vi "lorentzian transformations--test.vi"() -> ()   [LabVIEW 2020]
uses:
  lorentzian.ctl
  circle corners.ctl
  cursor action.ctl
  four-corner circle transformation.ctl
  draw a circle.vi
  draw a complex arrow.vi
  Q -- check range -- i -- real.vi
  generate linear region.vi
  draw a complex line.vi
  Q - not nan -- real.vi
panel:
  in  "Tab Control":enum32{"Page 1", "Page 2"}(tab)
  in  "phase0":dbl(slide)=-0.3274811506911865 scale=-1.57..1.57
  in  "factor":dbl(slide)=0.3 scale=-3.0..3.0
  in  "phase":dbl(slide)=-0.2854545454545454 scale=-1.57..1.57
  out "Plot: complex plane":cluster{dbl[], dbl[]}[](graph)=[{[1.005, 1.0049956141504943, 1.0049824642962475, 1.0049605735065723, 1.0049299801853526, 1.0048907380036691, 1.004842915805643, 1.0047865974876604, 1.0047218818511874, 1.0046488824294413, 1.004567727288213, 1.004478558801197, 1.0043815334002193, 1.0042768213008024, 1.0041646062035505, 1.0040450849718747, 1.0039184672866293, 1.0037849752782588, 1.003644843137107, 1.0034983167025668, 1.0033456530317943, 1.0031871199487434, 1.003022995574312, 1.002853567838422, 1.002679133974895, 1.0025, 1.0023164801755993, 1.0021288964578254, 1.0019375779322606, 1.001742860236609, 1.0015450849718748, 1.0013445991030763, 1.0011417543505532, 1.0009369065729286, 1.000730415142812, 1.0005226423163383, 1.0003139525976465, 1.0001047120994169, 0.9998952879005832, 0.9996860474023535, 0.9994773576836617, 0.999269584857188, 0.9990630934270713, 0.9988582456494467, 0.9986554008969236, 0.9984549150281252, 0.9982571397633909, 0.9980624220677395, 0.9978711035421747, 0.9976835198244007, 0.9975, 0.9973208660251051, 0.9971464321615778, 0.9969770044256882, 0.9968128800512566, 0.9966543469682058, 0.9965016832974332, 0.996355156862893, 0.9962150247217412, 0.9960815327133709, 0.9959549150281253, 0.9958353937964495, 0.9957231786991975, 0.9956184665997807, 0.9955214411988029, 0.995432272711787, 0.9953511175705587, 0.9952781181488126, 0.9952134025123397, 0.9951570841943569, 0.995109261996331, 0.9950700198146475, 0.9950394264934276, 0.9950175357037525, 0.9950043858495057, 0.995, 0.9950043858495057, 0.9950175357037525, 0.9950394264934276, 0.9950700198146475, 0.995109261996331, 0.9951570841943569, 0.9952134025123397, 0.9952781181488126, 0.9953511175705587, 0.995432272711787, 0.9955214411988029, 0.9956184665997807, 0.9957231786991975, 0.9958353937964495, 0.9959549150281253, 0.9960815327133709, 0.9962150247217412, 0.9963551568628929, 0.9965016832974332, 0.9966543469682058, 0.9968128800512566, 0.9969770044256882, 0.9971464321615778, 0.9973208660251051, 0.9975, 0.9976835198244007, 0.9978711035421747, 0.9980624220677394, 0.9982571397633909, 0.9984549150281252, 0.9986554008969236, 0.9988582456494467, 0.9990630934270713, 0.999269584857188, 0.9994773576836617, 0.9996860474023535, 0.9998952879005832, 1.0001047120994169, 1.0003139525976465, 1.0005226423163383, 1.000730415142812, 1.0009369065729286, 1.0011417543505532, 1.0013445991030763, 1.0015450849718748, 1.001742860236609, 1.0019375779322606, 1.0021288964578254, 1.0023164801755993, 1.0025, 1.002679133974895, 1.002853567838422, 1.003022995574312, 1.0031871199487434, 1.0033456530317943, 1.0034983167025668, 1.003644843137107, 1.0037849752782588, 1.0039184672866293, 1.0040450849718747, 1.0041646062035505, 1.0042768213008024, 1.0043815334002193, 1.004478558801197, 1.004567727288213, 1.0046488824294413, 1.0047218818511874, 1.0047865974876604, 1.004842915805643, 1.0048907380036691, 1.0049299801853526, 1.0049605735065723, 1.0049824642962475, 1.0049956141504943], [0.995, 0.995209378268646, 0.9954183892166616, 0.9956266661678215, 0.9958338437335805, 0.9960395584540888, 0.9962434494358243, 0.9964451589847223, 0.996644333233693, 0.9968406227634233, 0.997033683215379, 0.9972231758959247, 0.9974087683705086, 0.9975901350468657, 0.9977669577462167, 0.9979389262614624, 0.9981057389013915, 0.9982671030199505, 0.9984227355296434, 0.998572363398164, 0.998715724127387, 0.998852566213879, 0.998982649590121, 0.9991057460456685, 0.9992216396275101, 0.9993301270189222, 0.9994310178961561, 0.9995241352623301, 0.9996093157579425, 0.9996864099474595, 0.9997552825814757, 0.9998158128339882, 0.9998678945143658, 0.9999114362536434, 0.999946361664815, 0.9999726094768414, 0.9999901336421414, 0.9999989034173742, 0.9999989034173742, 0.9999901336421414, 0.9999726094768414, 0.999946361664815, 0.9999114362536434, 0.9998678945143658, 0.9998158128339882, 0.9997552825814757, 0.9996864099474595, 0.9996093157579425, 0.9995241352623301, 0.9994310178961561, 0.9993301270189222, 0.9992216396275101, 0.9991057460456685, 0.998982649590121, 0.998852566213879, 0.998715724127387, 0.998572363398164, 0.9984227355296434, 0.9982671030199505, 0.9981057389013915, 0.9979389262614624, 0.9977669577462167, 0.9975901350468657, 0.9974087683705086, 0.9972231758959247, 0.997033683215379, 0.9968406227634233, 0.996644333233693, 0.9964451589847223, 0.9962434494358243, 0.9960395584540888, 0.9958338437335805, 0.9956266661678215, 0.9954183892166616, 0.995209378268646, 0.995, 0.994790621731354, 0.9945816107833384, 0.9943733338321785, 0.9941661562664195, 0.9939604415459112, 0.9937565505641758, 0.9935548410152777, 0.993355666766307, 0.9931593772365767, 0.992966316784621, 0.9927768241040753, 0.9925912316294914, 0.9924098649531343, 0.9922330422537833, 0.9920610737385376, 0.9918942610986085, 0.9917328969800495, 0.9915772644703565, 0.991427636601836, 0.991284275872613, 0.991147433786121, 0.991017350409879, 0.9908942539543315, 0.9907783603724899, 0.9906698729810778, 0.9905689821038439, 0.9904758647376699, 0.9903906842420575, 0.9903135900525405, 0.9902447174185243, 0.9901841871660118, 0.9901321054856342, 0.9900885637463566, 0.990053638335185, 0.9900273905231586, 0.9900098663578586, 0.9900010965826258, 0.9900010965826258, 0.9900098663578586, 0.9900273905231586, 0.990053638335185, 0.9900885637463566, 0.9901321054856342, 0.9901841871660118, 0.9902447174185243, 0.9903135900525405, 0.9903906842420575, 0.9904758647376699, 0.9905689821038439, 0.9906698729810778, 0.9907783603724899, 0.9908942539543315, 0.991017350409879, 0.991147433786121, 0.991284275872613, 0.991427636601836, 0.9915772644703565, 0.9917328969800495, 0.9918942610986085, 0.9920610737385376, 0.9922330422537833, 0.9924098649531343, 0.9925912316294914, 0.9927768241040753, 0.992966316784621, 0.9931593772365767, 0.993355666766307, 0.9935548410152777, 0.9937565505641757, 0.9939604415459112, 0.9941661562664195, 0.9943733338321785, 0.9945816107833384, 0.994790621731354]}, {[1.0, 1.0, 1.0, 1.0, 1.0, 1.0, 1.0, 1.0, 1.0, 1.0, 1.0, 1.0, 1.0, 1.0, 1.0, 1.0, 1.0, 1.0, 1.0, 1.0], [1.0, 0.9995, 0.999, 0.9984999999999999, 0.998, 0.9975, 0.997, 0.9964999999999999, 0.996, 0.9955, 0.995, 0.9944999999999999, 0.994, 0.9935, 0.993, 0.9924999999999999, 0.992, 0.9915, 0.991, 0.9904999999999999]}, {[1.005, 1.0045, 1.004, 1.0034999999999998, 1.003, 1.0025, 1.002, 1.0014999999999998, 1.001, 1.0005, 1.0, 0.9994999999999999, 0.999, 0.9984999999999999, 0.998, 0.9974999999999999, 0.997, 0.9964999999999999, 0.996, 0.9954999999999999], [0.995, 0.995, 0.995, 0.995, 0.995, 0.995, 0.995, 0.995, 0.995, 0.995, 0.995, 0.995, 0.995, 0.995, 0.995, 0.995, 0.995, 0.995, 0.995, 0.995]}, {[1.01, 1.009, 1.008, 1.0070000000000001, 1.006, 1.005, 1.004, 1.0030000000000001, 1.002, 1.001, 1.0, 0.999, 0.998, 0.997, 0.996, 0.995, 0.994, 0.993, 0.992, 0.991], [1.0, 1.0, 1.0, 1.0, 1.0, 1.0, 1.0, 1.0, 1.0, 1.0, 1.0, 1.0, 1.0, 1.0, 1.0, 1.0, 1.0, 1.0, 1.0, 1.0]}, {[1.0059232929877608, 1.0059187898532358, 1.0059052883496888, 1.005882812163345, 1.0058514007250723, 1.0058111091412076, 1.0057620080968799, 1.0057041837320058, 1.00563773749017, 1.005562785940659, 1.0054794605739599, 1.0053879075710797, 1.0052882875470954, 1.0051807752693802, 1.0050655593510023, 1.0049428419198327, 1.0048128382639459, 1.0046757764539296, 1.0045318969427723, 1.0043814521440277, 1.0042247059889937, 1.0040619334636893, 1.003893420126434, 1.003719461606883, 1.003540363087391, 1.0033564387676188, 1.003168011313322, 1.0029754112902827, 1.0027789765843875, 1.00257905180886, 1.0023759876996907, 1.0021701405003292, 1.00196187133671, 1.0017515455837172, 1.00153953222419, 1.001326203201604, 1.0011119327675542, 1.000897096825192, 1.0006820722697616, 1.0004672363273994, 1.0002529658933497, 1.0000396368707636, 0.9998276235112366, 0.9996172977582435, 0.9994090285946245, 0.9992031813952629, 0.9990001172860937, 0.998800192510566, 0.998603757804671, 0.9984111577816318, 0.9982227303273348, 0.9980388060075627, 0.9978597074880705, 0.9976857489685195, 0.9975172356312644, 0.9973544631059599, 0.997197716950926, 0.9970472721521811, 0.996903392641024, 0.9967663308310076, 0.9966363271751209, 0.9965136097439514, 0.9963983938255734, 0.9962908815478583, 0.9961912615238739, 0.9960997085209937, 0.9960163831542945, 0.9959414316047838, 0.9958749853629478, 0.9958171609980736, 0.995768059953746, 0.9957277683698812, 0.9956963569316087, 0.9956738807452647, 0.9956603792417177, 0.9956558761071926, 0.9956603792417177, 0.9956738807452647, 0.9956963569316087, 0.9957277683698812, 0.995768059953746, 0.9958171609980736, 0.9958749853629478, 0.9959414316047838, 0.9960163831542945, 0.9960997085209937, 0.9961912615238739, 0.9962908815478583, 0.9963983938255734, 0.9965136097439514, 0.9966363271751209, 0.9967663308310076, 0.996903392641024, 0.9970472721521811, 0.997197716950926, 0.9973544631059599, 0.9975172356312644, 0.9976857489685195, 0.9978597074880705, 0.9980388060075627, 0.9982227303273348, 0.9984111577816318, 0.998603757804671, 0.998800192510566, 0.9990001172860937, 0.9992031813952629, 0.9994090285946245, 0.9996172977582435, 0.9998276235112366, 1.0000396368707636, 1.0002529658933497, 1.0004672363273994, 1.0006820722697616, 1.000897096825192, 1.0011119327675542, 1.001326203201604, 1.00153953222419, 1.0017515455837172, 1.00196187133671, 1.0021701405003292, 1.0023759876996907, 1.00257905180886, 1.0027789765843875, 1.0029754112902827, 1.003168011313322, 1.0033564387676188, 1.003540363087391, 1.003719461606883, 1.003893420126434, 1.0040619334636893, 1.0042247059889937, 1.0043814521440277, 1.0045318969427723, 1.0046757764539296, 1.0048128382639459, 1.0049428419198327, 1.005065559351002, 1.0051807752693802, 1.0052882875470954, 1.0053879075710797, 1.0054794605739599, 1.005562785940659, 1.00563773749017, 1.0057041837320058, 1.0057620080968799, 1.0058111091412076, 1.0058514007250723, 1.005882812163345, 1.0059052883496888, 1.0059187898532358], [0.994938915988178, 0.99515389338517, 0.9953684936387578, 0.9955823402671752, 0.9957950581107701, 0.9960062739901628, 0.9962156173609295, 0.9964227209636622, 0.9966272214682678, 0.9968287601113711, 0.997026983325709, 0.9972215433604069, 0.9974120988910519, 0.997598315618492, 0.9977798668553104, 0.9979564340989464, 0.9981277075904564, 0.9982933868579376, 0.9984531812436561, 0.9986068104139613, 0.9987540048510848, 0.9988945063259668, 0.9990280683512777, 0.9991544566138403, 0.9992734493856953, 0.9993848379130866, 0.9994884267826872, 0.9995840342644202, 0.9996714926302748, 0.9997506484485588, 0.9998213628530697, 0.9998835117867129, 0.9999369862191405, 0.9999816923380274, 1.0000175517136496, 1.0000445014364774, 1.0000624942275393, 1.000071498521366, 1.000071498521366, 1.0000624942275393, 1.0000445014364774, 1.0000175517136496, 0.9999816923380274, 0.9999369862191405, 0.9998835117867129, 0.9998213628530697, 0.9997506484485588, 0.9996714926302748, 0.9995840342644202, 0.9994884267826872, 0.9993848379130866, 0.9992734493856953, 0.9991544566138403, 0.9990280683512777, 0.9988945063259668, 0.9987540048510848, 0.9986068104139613, 0.9984531812436561, 0.9982933868579376, 0.9981277075904564, 0.9979564340989464, 0.9977798668553104, 0.997598315618492, 0.9974120988910519, 0.9972215433604069, 0.997026983325709, 0.9968287601113711, 0.9966272214682678, 0.9964227209636622, 0.9962156173609295, 0.9960062739901628, 0.9957950581107701, 0.9955823402671752, 0.9953684936387579, 0.99515389338517, 0.994938915988178, 0.9947239385911859, 0.9945093383375981, 0.9942954917091807, 0.9940827738655859, 0.9938715579861931, 0.9936622146154265, 0.9934551110126937, 0.9932506105080882, 0.9930490718649848, 0.9928508486506469, 0.992656288615949, 0.9924657330853041, 0.9922795163578639, 0.9920979651210455, 0.9919213978774095, 0.9917501243858995, 0.9915844451184184, 0.9914246507326998, 0.9912710215623947, 0.9911238271252711, 0.9909833256503892, 0.9908497636250783, 0.9907233753625156, 0.9906043825906606, 0.9904929940632693, 0.9903894051936687, 0.9902937977119357, 0.9902063393460812, 0.9901271835277972, 0.9900564691232863, 0.9899943201896431, 0.9899408457572154, 0.9898961396383286, 0.9898602802627063, 0.9898333305398784, 0.9898153377488166, 0.9898063334549901, 0.9898063334549901, 0.9898153377488166, 0.9898333305398784, 0.9898602802627063, 0.9898961396383286, 0.9899408457572154, 0.9899943201896431, 0.9900564691232863, 0.9901271835277972, 0.9902063393460812, 0.9902937977119357, 0.9903894051936687, 0.9904929940632693, 0.9906043825906606, 0.9907233753625156, 0.9908497636250783, 0.9909833256503892, 0.9911238271252711, 0.9912710215623947, 0.9914246507326998, 0.9915844451184184, 0.9917501243858995, 0.9919213978774095, 0.9920979651210455, 0.9922795163578639, 0.9924657330853041, 0.992656288615949, 0.9928508486506469, 0.9930490718649848, 0.9932506105080882, 0.9934551110126937, 0.9936622146154265, 0.9938715579861931, 0.9940827738655859, 0.9942954917091807, 0.994509338337598, 0.9947239385911859]}, {[1.0007895845474768, 1.0007895845474768, 1.0007895845474768, 1.0007895845474768, 1.0007895845474768, 1.0007895845474768, 1.0007895845474768, 1.0007895845474768, 1.0007895845474768, 1.0007895845474768, 1.0007895845474768, 1.0007895845474768, 1.0007895845474768, 1.0007895845474768, 1.0007895845474768, 1.0007895845474768, 1.0007895845474768, 1.0007895845474768, 1.0007895845474768, 1.0007895845474768], [1.0000726244284621, 0.9995592535844338, 0.9990458827404053, 0.9985325118963768, 0.9980191410523485, 0.9975057702083201, 0.9969923993642916, 0.9964790285202632, 0.9959656576762348, 0.9954522868322064, 0.994938915988178, 0.9944255451441495, 0.9939121743001211, 0.9933988034560928, 0.9928854326120643, 0.9923720617680358, 0.9918586909240075, 0.9913453200799791, 0.9908319492359506, 0.9903185783919222]}, {[1.0059232929877608, 1.0054099221437325, 1.0048965512997041, 1.0043831804556755, 1.0038698096116472, 1.0033564387676188, 1.0028430679235905, 1.0023296970795619, 1.0018163262355335, 1.0013029553915052, 1.0007895845474768, 1.0002762137034484, 0.99976284285942, 0.9992494720153915, 0.9987361011713631, 0.9982227303273347, 0.9977093594833063, 0.9971959886392778, 0.9966826177952495, 0.996169246951221], [0.994938915988178, 0.994938915988178, 0.994938915988178, 0.994938915988178, 0.994938915988178, 0.994938915988178, 0.994938915988178, 0.994938915988178, 0.994938915988178, 0.994938915988178, 0.994938915988178, 0.994938915988178, 0.994938915988178, 0.994938915988178, 0.994938915988178, 0.994938915988178, 0.994938915988178, 0.994938915988178, 0.994938915988178, 0.994938915988178]}, {[1.011057001428045, 1.0100302597399882, 1.0090035180519314, 1.0079767763638747, 1.0069500346758178, 1.0059232929877608, 1.0048965512997041, 1.0038698096116474, 1.0028430679235905, 1.0018163262355335, 1.0007895845474768, 0.99976284285942, 0.9987361011713631, 0.9977093594833063, 0.9966826177952495, 0.9956558761071926, 0.9946291344191358, 0.993602392731079, 0.9925756510430221, 0.9915489093549653], [1.0000726244284621, 1.0000726244284621, 1.0000726244284621, 1.0000726244284621, 1.0000726244284621, 1.0000726244284621, 1.0000726244284621, 1.0000726244284621, 1.0000726244284621, 1.0000726244284621, 1.0000726244284621, 1.0000726244284621, 1.0000726244284621, 1.0000726244284621, 1.0000726244284621, 1.0000726244284621, 1.0000726244284621, 1.0000726244284621, 1.0000726244284621, 1.0000726244284621]}]
  in  "lorentzian":T1={"A (VHz)"=1.0, "f (Hz)"=900.0, "G (Hz)"=200.0, "phi(rad)"=0.0, "Q"=0.006429595340103388, "Norm  Ampl"=nan, "bg (V)"=1.0+1.0i, "4corners"={"z (-pi/2)"=1.005+0.995i, "z(inf)"=1.0+1.0i, "z (pi/2)"=0.995+0.995i, "z center"=1.0+0.995i, "z(0)"=1.0+0.99i, "radius"=0.005}} {"bg (V)" format="%#9_9f"; "Q" format="%#9_9f"; "phi(rad)" format="%#9_9f"; "G (Hz)" format="%#9_9f"; "f (Hz)" format="%#9_9f"}
  in  "exit":bool
  in  "omega":dbl(slide)=866.0287081339713 scale=500.0..1500.0
  in  "lorentzian hist":T1={"A (VHz)"=1.0, "f (Hz)"=892.9671519759877, "G (Hz)"=194.7909608876527, "phi(rad)"=0.0, "Q"=0.006429595340103388, "Norm  Ampl"=nan, "bg (V)"=1.0007895845474768+1.0000726244284621i, "4corners"={"z (-pi/2)"=1.0059232929877608+0.994938915988178i, "z(inf)"=1.0007895845474768+1.0000726244284621i, "z (pi/2)"=0.9956558761071926+0.994938915988178i, "z center"=1.0007895845474768+0.994938915988178i, "z(0)"=1.0007895845474768+0.9898052075478938i, "radius"=0.005133708440284138}} {"bg (V)" format="%#9_9f"; "Q" format="%#9_9f"; "phi(rad)" format="%#9_9f"; "G (Hz)" format="%#9_9f"; "f (Hz)" format="%#9_9f"}
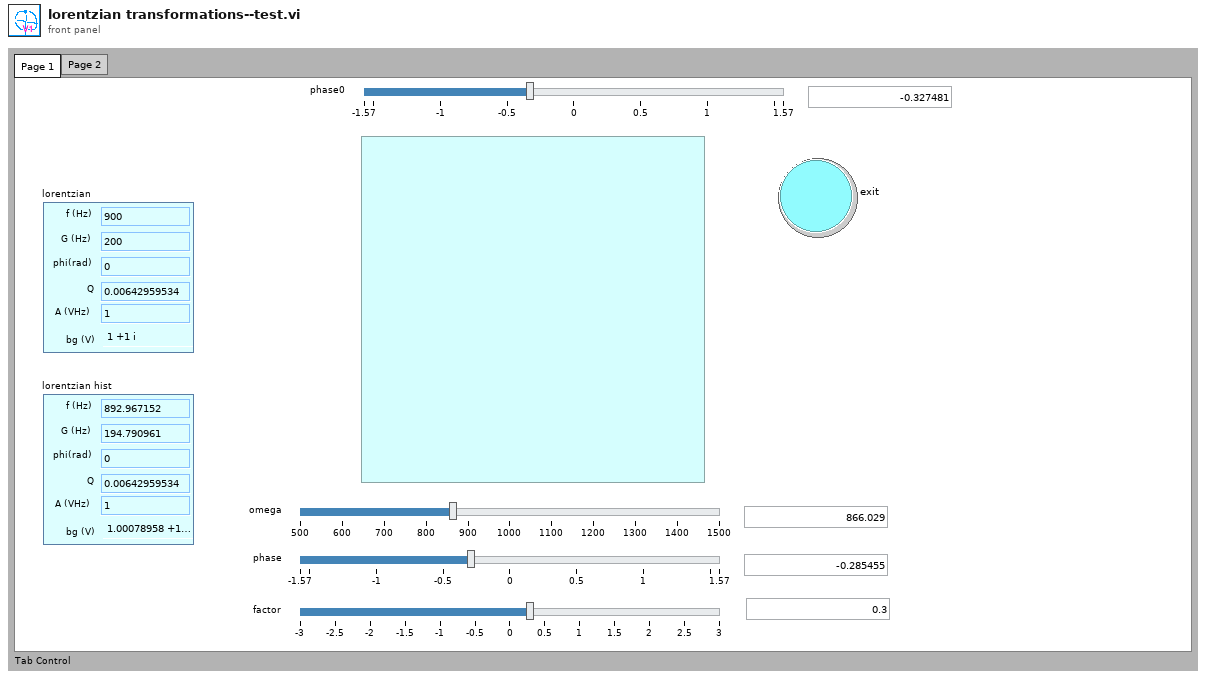
[diagram p1: front panel]
types:
  T1 = typedef "lorentzian.ctl" = cluster{"A (VHz)":dbl, "f (Hz)":dbl, "G (Hz)":dbl, "phi(rad)":dbl, "Q":dbl, "Norm  Ampl":dbl, "bg (V)":cdb, "4corners":T2}
  T2 = typedef "circle corners.ctl" = cluster{"z (-pi/2)":cdb, "z(inf)":cdb, "z (pi/2)":cdb, "z center":cdb, "z(0)":cdb, "radius":dbl}
  T3 = typedef "cursor action.ctl" = enum16{"range", "read", "write", "check", "zoom out", "smart zoom out", "zoom to aspect ratio 1", "zoom to win", "zoom out 20%", "zoom in 20%", "-empty", "smart zoom out&aspect", "move range left 20%", "move range right 20%", "move range up 20%", "move range down 20%", "zoom to X win", "zoom to Y win", "zoom out X", "zoom out Y", "zoom in X", "zoom in Y", "check plot scale"}
  T4 = typedef "eventvkey.ctl" = enum16{"ASCII", "Enter", "Return", "Shift", "Ctrl", "Alt", "Cmd", "Opt", "Caps", "NumLock", "Clear", "Break", "Up", "Down", "Left", "Right", "Insert", "Delete", "Home", "End", "PageUp", "PageDown", "Escape", "Help", "Pause", "ScrollLock", "F1", "F2", "F3", "F4", "F5", "F6", "F7", "F8", "F9", "F10", "F11", "F12", "F13", "F14", "F15", "F16", "F17", "F18", "F19", "F20", "F21", "F22", "F23", "F24", "Play", "VolumeUp", "VolumeDown", "Mute", "Two Byte Char"}
  T5 = typedef "four-corner circle transformation.ctl" = enum16{"z(c) z(inf)", "z(c) z(zero)", "fix phase", "calculate lorentzian", "z(0) z(+-pi/2)", "shift to zcenter", "to  canonical", "get canonical phase", "get4corners", "update lorentzian -- from z0", "fake gamma normal", "fake gamma heat", "calculate complex slope", "get f0 given f and phi"}
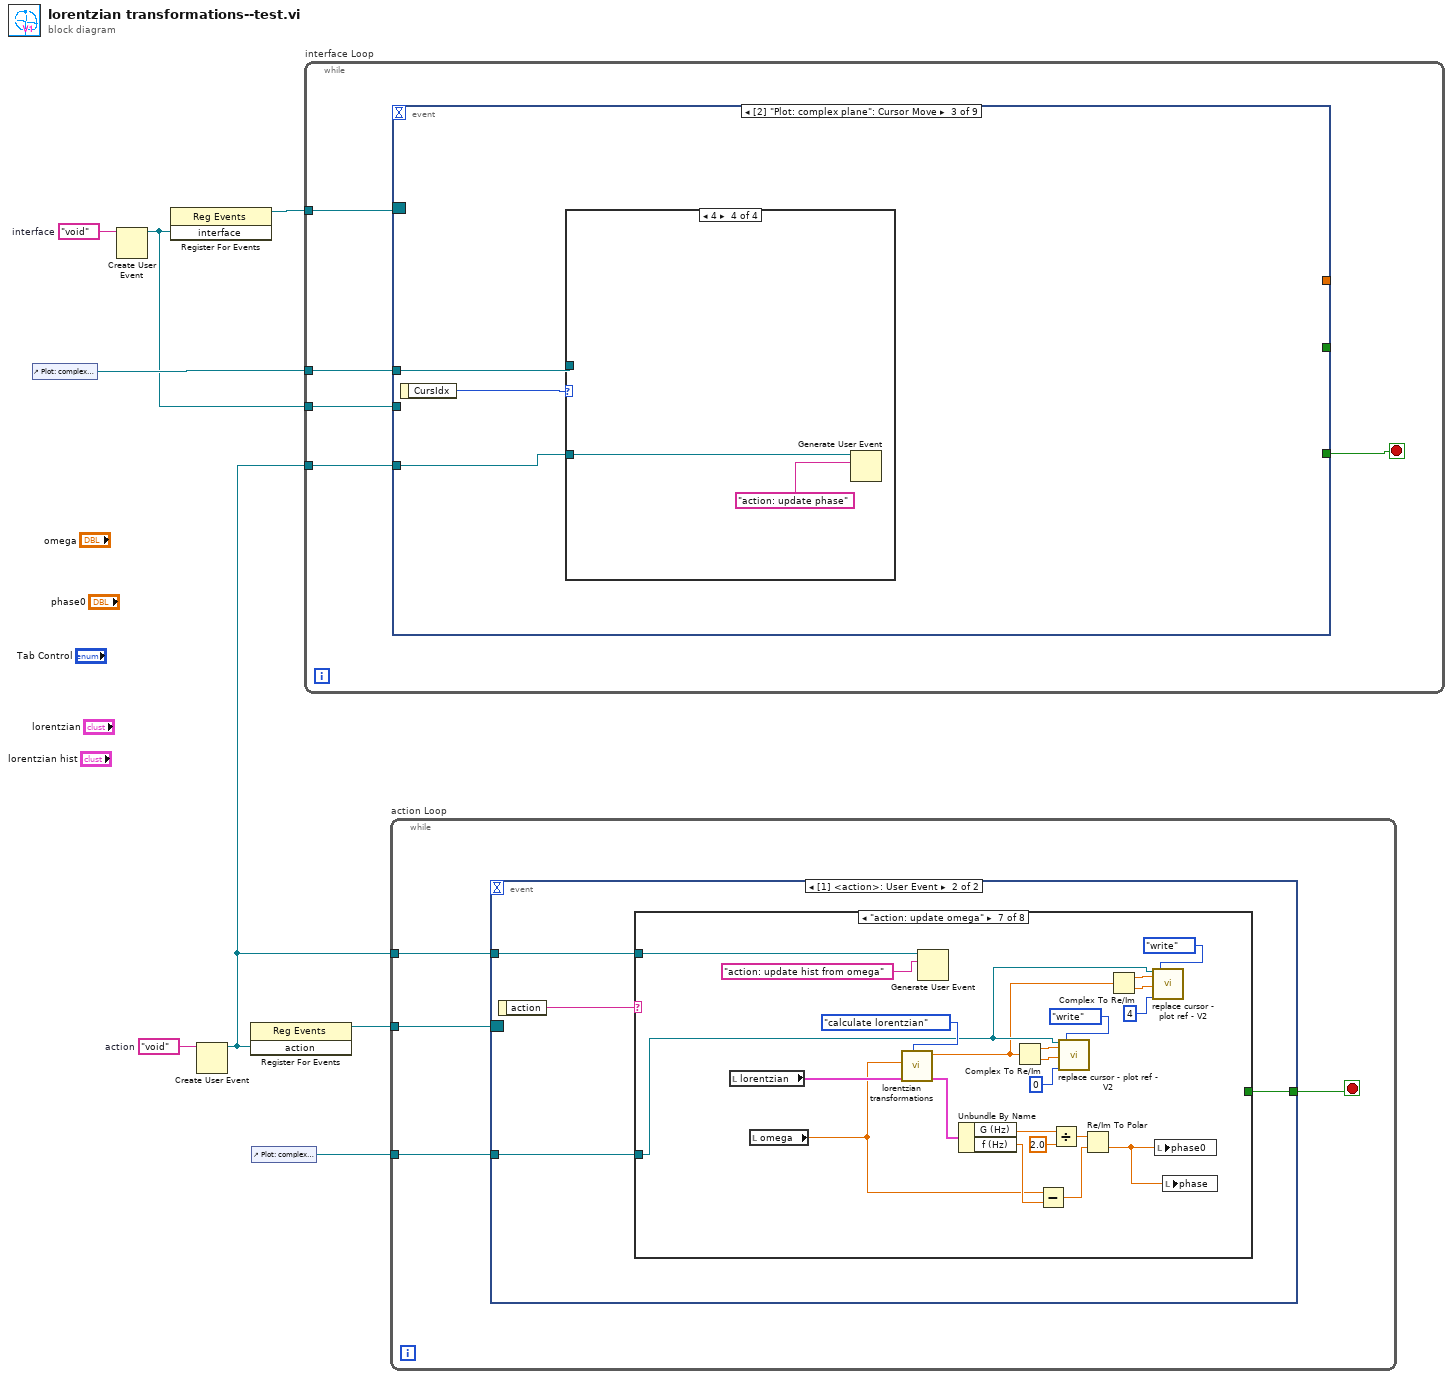
[diagram p0: block diagram]
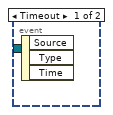
[diagram p2: hidden frame]
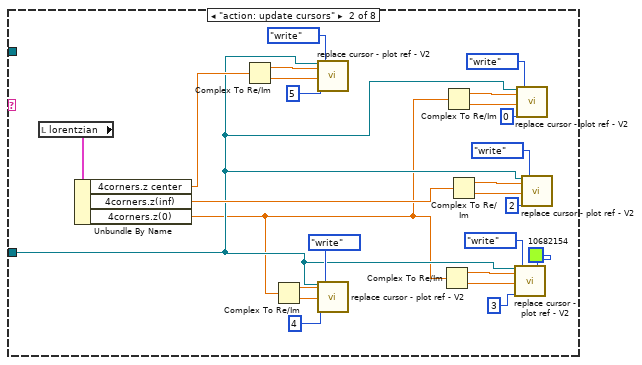
[diagram p4: hidden frame]
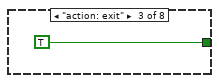
[diagram p5: hidden frame]
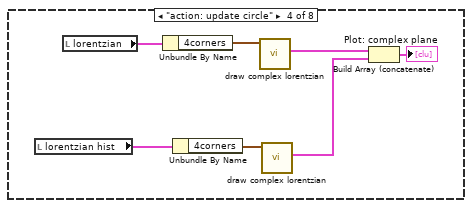
[diagram p6: hidden frame]
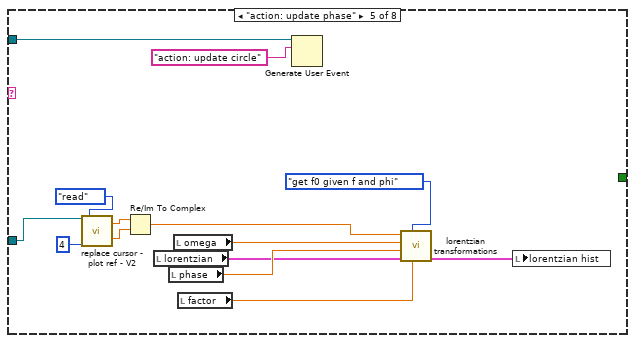
[diagram p7: hidden frame]
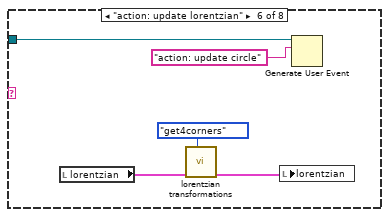
[diagram p8: hidden frame]
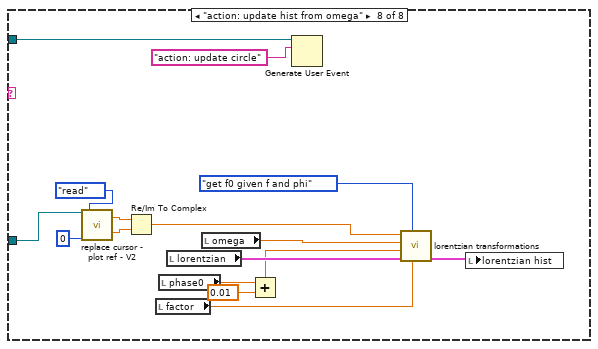
[diagram p9: hidden frame]
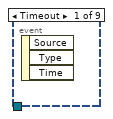
[diagram p10: hidden frame]
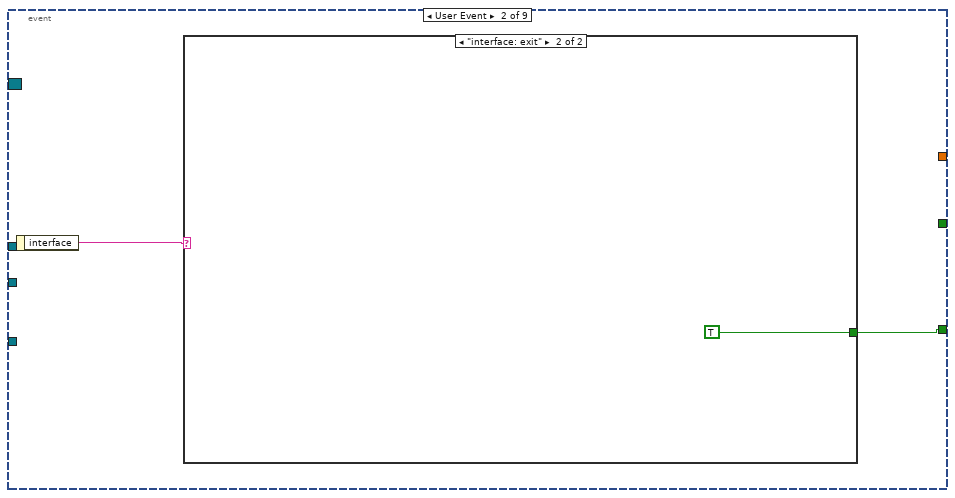
[diagram p11: hidden frame]
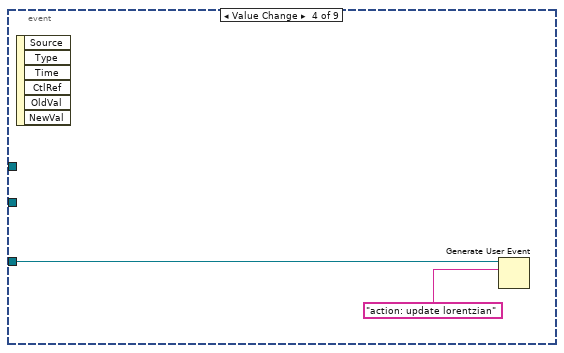
[diagram p16: hidden frame]
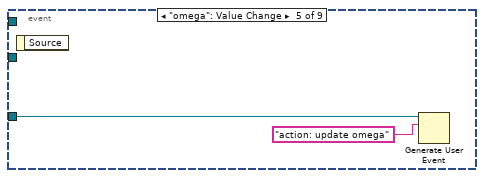
[diagram p17: hidden frame]
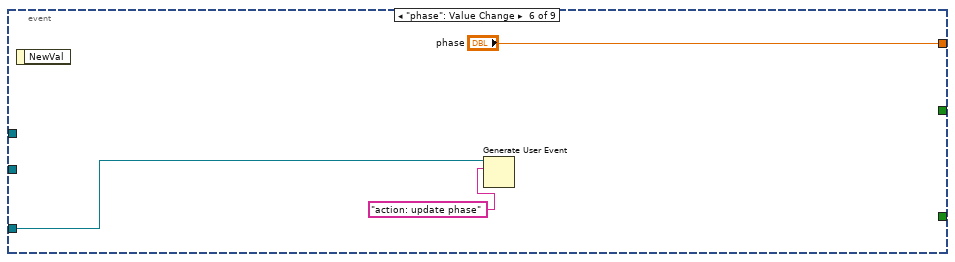
[diagram p18: hidden frame]
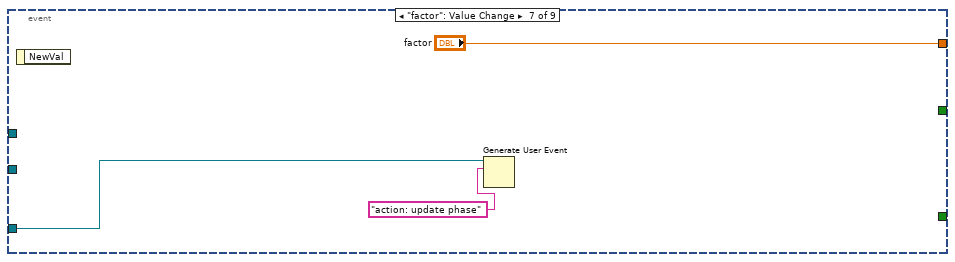
[diagram p19: hidden frame]
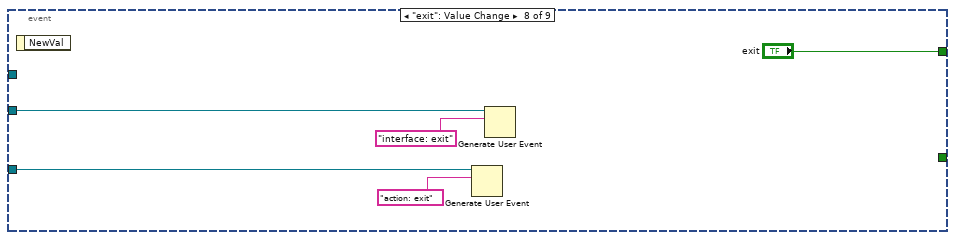
[diagram p20: hidden frame]
diagram:
  w5 = "void"  # interface
  w8 = "void"  # action
  n1 = control-ref of="Plot: complex plane"() -> (w3:refnum<vi>)
  n2 = Create User Event(user event datatype=w5) -> (user event=w2:refnum<user-event>)  [unwired: 1 in, 1 out]
  n3 = register-events(w2) -> (reference out=w4:refnum<event-registration>)  [unwired: 2 in, 1 out]
  n4 = Create User Event(user event datatype=w8) -> (user event=w1:refnum<user-event>)  [unwired: 1 in, 1 out]
  n5 = register-events(w1) -> (reference out=w7:refnum<event-registration>)  [unwired: 2 in, 1 out]
  n6 = control-ref of="Plot: complex plane"() -> (w6:refnum<vi>)
  n7 = while "interface Loop" {
    tunnel: w4 -> [w13]
    tunnel: w1 -> [w12]
    tunnel: w3 -> [w11]
    tunnel: w2 -> [w9]
    stop <- w10 stop-if-true
    n8 = event shown="[2] \"Plot: complex plane\": Cursor Move" {
      selector: w13 -> [_ _ _ _ _ _ _ _ _]
      dyn-events: _ -> [_ _ _ _ _ _ _ _ _]
      timeout: _ -> [_ _ _ _ _ _ _ _ _]
      tunnel: [_ _ _ _ _ _ _ "exit" _] -> _
      tunnel: w12 -> [_ _ w17 w22 w24 w26 w30 w34 w37]
      tunnel: w11 -> [_ _ w19 _ _ _ _ _ w38]
      tunnel: [_ w14 _ _ _ _ _ _ _] -> w10
      tunnel: w9 -> [_ _ _ _ _ _ _ w32 _]
      tunnel: [_ _ _ _ _ "phase" "factor" _ _] -> _
      event Timeout {
        n9 = event-data() -> ()  [unwired: 1 in, 3 out]
      }
      event User Event {
        n10 = event-data() -> ("interface"=w15:string)  [unwired: 1 in]
        n11 = case shown="\"interface: exit\"" w15 {
          tunnel: [_ TRUE] -> w14
          frame "False", Default {
          }
          frame "interface: exit" {
          }
        }
      }
      event "Plot: complex plane": Cursor Move {
        n12 = event-data() -> ("CursIdx"=w18:i32)  [unwired: 1 in]
        n13 = case shown="4" w18 {
          tunnel: w19 -> [_ _ _ _]
          tunnel: w17 -> [_ _ _ w20]
          frame 0, Default {
          }
          frame 2 {
          }
          frame 3 {
          }
          frame 4 {
            n14 = Generate User Event(user event=w20, event data cluster="action: update phase" ("event data")) -> ()  [unwired: 2 in, 2 out]
          }
        }
      }
      event Value Change {
        n15 = event-data() -> ()  [unwired: 1 in, 6 out]
        n16 = Generate User Event(user event=w22, event data cluster="action: update lorentzian" ("event data")) -> ()  [unwired: 2 in, 2 out]
      }
      event "omega": Value Change {
        n17 = event-data() -> ()  [unwired: 1 in, 1 out]
        n18 = Generate User Event(user event=w24, event data cluster="action: update omega" ("event data")) -> ()  [unwired: 2 in, 2 out]
      }
      event "phase": Value Change {
        n19 = event-data() -> ()  [unwired: 1 in, 1 out]
        n20 = Generate User Event(user event=w26, event data cluster="action: update phase" ("event data")) -> ()  [unwired: 2 in, 2 out]
      }
      event "factor": Value Change {
        n21 = event-data() -> ()  [unwired: 1 in, 1 out]
        n22 = Generate User Event(user event=w30, event data cluster="action: update phase" ("event data")) -> ()  [unwired: 2 in, 2 out]
      }
      event "exit": Value Change {
        n23 = event-data() -> ()  [unwired: 1 in, 1 out]
        n24 = Generate User Event(user event=w34, event data cluster="action: exit" ("event data")) -> ()  [unwired: 2 in, 2 out]
        n25 = Generate User Event(user event=w32, event data cluster="interface: exit" ("event data")) -> ()  [unwired: 2 in, 2 out]
      }
      event Key Down {
        n26 = event-data() -> ("VKey"=w40:T4, "Char"=w39:i16)  [unwired: 1 in]
        n27 = Build Array(w39) -> (w42:i16[])
        n28 = Byte Array To String(unsigned byte array=w42) -> (string=w41:string)
        n29 = case shown="\"ASCII\", Default" w40 {
          selector: w40 -> [_ _ _ _ w58]
          tunnel: w39 -> [_ _ _ _ _]
          tunnel: w41 -> [w45 _ _ _ _]
          tunnel: w38 -> [w44 _ _ _ w56]
          tunnel: w37 -> [w43 _ _ _ _]
          frame "ASCII", Default {
            n30 = case shown="\" \"" w45 {
              selector: w45 -> [_ w47 _ _ _ _ _]
              tunnel: w44 -> [_ w46 _ _ _ _ _]
              tunnel: w43 -> [_ _ w54 _ _ _ _]
              frame "0", Default {
              }
              frame "<", ">", "?", "A", "z" {
                n31 = case shown="\"?\"" w47 {
                  tunnel: [cursor_action."zoom out 20%" ("cursor action") cursor_action."zoom in 20%" ("cursor action") cursor_action."smart zoom out&aspect" ("cursor action") cursor_action."smart zoom out" ("cursor action") cursor_action."zoom to aspect ratio 1" ("cursor action")] -> w48
                  frame ">" {
                  }
                  frame "<" {
                  }
                  frame "?" {
                  }
                  frame "A" {
                  }
                  frame "z", Default {
                  }
                }
                n32 = call "replace cursor - plot ref - V2.vi"("Plot ref in"=w46, "cursor action"=w48) -> ()  [unwired: 14 in, 4 out]
                n33 = call "replace cursor - plot ref - V2.vi"("Plot ref in"=w46, "cursor action"=w48) -> ()  [unwired: 14 in, 4 out]
              }
              frame " " {
                n34 = Generate User Event(user event=w54, event data cluster="action: update cursors" ("event data")) -> ()  [unwired: 2 in, 2 out]
              }
              frame "'", ";", "[", "]", "{", "}" {
              }
              frame "@" {
              }
              frame "#" {
              }
              frame "q" {
              }
            }
          }
          frame "Escape" {
          }
          frame "PageUp" {
          }
          frame "PageDown" {
          }
          frame "Up".."Right" {
            n35 = case shown="\"Down\"" w58 {
              tunnel: [cursor_action."move range right 20%" ("cursor action") cursor_action."move range left 20%" ("cursor action") cursor_action."move range up 20%" ("cursor action") cursor_action."move range down 20%" ("cursor action")] -> w57
              frame "Right", Default {
              }
              frame "Left" {
              }
              frame "Up" {
              }
              frame "Down" {
              }
            }
            n36 = call "replace cursor - plot ref - V2.vi"("Plot ref in"=w56, "cursor action"=w57) -> ()  [unwired: 14 in, 4 out]
            n37 = call "replace cursor - plot ref - V2.vi"("Plot ref in"=w56, "cursor action"=w57) -> ()  [unwired: 14 in, 4 out]
          }
        }
      }
    }
  }
  n38 = while "action Loop" {
    tunnel: w7 -> [w66]
    tunnel: w6 -> [w65]
    tunnel: w1 -> [w63]
    stop <- w64 stop-if-true
    n39 = event shown="[1] <action>: User Event" {
      selector: w66 -> [_ _]
      dyn-events: _ -> [_ _]
      timeout: _ -> [_ _]
      tunnel: w65 -> [_ w69]
      tunnel: [_ w68] -> w64
      tunnel: w63 -> [_ w67]
      event Timeout {
        n40 = event-data() -> ()  [unwired: 1 in, 3 out]
      }
      event User Event {
        n41 = event-data() -> ("action"=w70:string)  [unwired: 1 in]
        n42 = case shown="\"action: update omega\"" w70 {
          tunnel: w69 -> [_ w72 _ _ w108 _ w125 w150]
          tunnel: [_ _ TRUE _ _ _ _ _] -> w68
          tunnel: w67 -> [_ _ _ _ w109 w122 w143 w151]
          frame "False", Default {
          }
          frame "action: update cursors" {
            n43 = local read "lorentzian"() -> (w77:T1)
            n44 = Unbundle By Name(w77) -> ("4corners.z center"=w78:cdb, "4corners.z(inf)"=w79:cdb, "4corners.z(0)"=w71:cdb)
            n45 = Complex To Re/Im(x + iy=w78) -> (x=w82:dbl, y=w83:dbl)
            n46 = Complex To Re/Im(x + iy=w71) -> (x=w87:dbl, y=w86:dbl)
            n47 = call "replace cursor - plot ref - V2.vi"("Plot ref in"=w72, "new X"=w82, "new  Y"=w83, "cursor index"=5, "cursor action"=cursor_action."write") -> ()  [unwired: 11 in, 4 out]
            n48 = call "replace cursor - plot ref - V2.vi"("Plot ref in"=w72, "new X"=w87, "new  Y"=w86, "cursor index"=4, "cursor action"=cursor_action."write") -> ()  [unwired: 11 in, 4 out]
            n49 = Complex To Re/Im(x + iy=w71) -> (x=w95:dbl, y=w96:dbl)
            n50 = Complex To Re/Im(x + iy=w71) -> (x=w75:dbl, y=w76:dbl)
            n51 = Complex To Re/Im(x + iy=w79) -> (x=w93:dbl, y=w94:dbl)
            n52 = call "replace cursor - plot ref - V2.vi"("Plot ref in"=w72, "new X"=w95, "new  Y"=w96, "cursor index"=3, "cursor action"=cursor_action."write", "Color Box"=u32 10682154) -> ()  [unwired: 10 in, 4 out]
            n53 = call "replace cursor - plot ref - V2.vi"("Plot ref in"=w72, "new X"=w75, "new  Y"=w76, "cursor index"=0, "cursor action"=cursor_action."write") -> ()  [unwired: 11 in, 4 out]
            n54 = call "replace cursor - plot ref - V2.vi"("Plot ref in"=w72, "new X"=w93, "new  Y"=w94, "cursor index"=2, "cursor action"=cursor_action."write") -> ()  [unwired: 11 in, 4 out]
          }
          frame "action: exit" {
          }
          frame "action: update circle" {
            n55 = local read "lorentzian hist"() -> (w99:T1)
            n56 = local read "lorentzian"() -> (w98:T1)
            n57 = Unbundle By Name(w98) -> ("4corners"=w104:T2)
            n58 = Unbundle By Name(w99) -> ("4corners"=w103:T2)
            n59 = call "draw complex lorentzian.vi"("4 corners"=w104) -> ("fancy circles"=w102:cluster{dbl[], dbl[]}[])  [unwired: 10 in]
            n60 = call "draw complex lorentzian.vi"("4 corners"=w103) -> ("fancy circles"=w101:cluster{dbl[], dbl[]}[])  [unwired: 10 in]
            n61 = Build Array (concatenate)(w102, w101) -> (→"Plot: complex plane":cluster{dbl[], dbl[]}[])
          }
          frame "action: update phase" {
            n62 = call "replace cursor - plot ref - V2.vi"("Plot ref in"=w108, "cursor index"=4, "cursor action"=cursor_action."read") -> ("read X"=w116:dbl, "read Y"=w115:dbl)  [unwired: 13 in, 2 out]
            n63 = Re/Im To Complex(1:w115, 2:w116) -> (0:w117:cdb)
            n64 = local read "lorentzian"() -> (w105:T1)
            n65 = local read "phase"() -> (w107:dbl)
            n66 = local read "omega"() -> (w114:dbl)
            n67 = local read "factor"() -> (w106:dbl)
            n68 = Generate User Event(user event=w109, event data cluster="action: update circle" ("event data")) -> ()  [unwired: 2 in, 2 out]
            n69 = call "lorentzian transformations.vi"("factor"=w106, "4 corner circle transformation"=four-corner_circle_transformation."get f0 given f and phi", "lorentzian in"=w105, "phase in (rad)"=w107, "freq in"=w114, "voltage in"=w117) -> ("lorentzian out"=w118:T1)  [unwired: 2 in, 3 out]
            n70 = local write "lorentzian hist"(w118) -> ()
          }
          frame "action: update lorentzian" {
            n71 = local read "lorentzian"() -> (w121:T1)
            n72 = call "lorentzian transformations.vi"("4 corner circle transformation"=four-corner_circle_transformation."get4corners", "lorentzian in"=w121) -> ("lorentzian out"=w119:T1)  [unwired: 6 in, 3 out]
            n73 = local write "lorentzian"(w119) -> ()
            n74 = Generate User Event(user event=w122, event data cluster="action: update circle" ("event data")) -> ()  [unwired: 2 in, 2 out]
          }
          frame "action: update omega" {
            n75 = local read "lorentzian"() -> (w138:T1)
            n76 = local read "omega"() -> (w131:dbl)
            n77 = call "lorentzian transformations.vi"("4 corner circle transformation"=four-corner_circle_transformation."calculate lorentzian", "lorentzian in"=w138, "freq in"=w131) -> ("voltage out"=w124:cdb)  [unwired: 5 in, 3 out]
            n78 = Generate User Event(user event=w143, event data cluster="action: update hist from omega" ("event data")) -> ()  [unwired: 2 in, 2 out]
            n79 = Unbundle By Name(w138) -> ("G (Hz)"=w139:dbl, "f (Hz)"=w141:dbl)
            n80 = Complex To Re/Im(x + iy=w124) -> (x=w136:dbl, y=w137:dbl)
            n81 = Subtract(x=w131, y=w141) -> (x-y=w142:dbl)
            n82 = Divide(x=w139, y=2.0) -> (x/y=w140:dbl)
            n83 = call "replace cursor - plot ref - V2.vi"("Plot ref in"=w125, "new X"=w136, "new  Y"=w137, "cursor index"=0, "cursor action"=cursor_action."write") -> ()  [unwired: 11 in, 4 out]
            n84 = Re/Im To Polar(2:w142, 3:w140) -> (0:w130:dbl)  [unwired: 1 out]
            n85 = Complex To Re/Im(x + iy=w124) -> (x=w128:dbl, y=w129:dbl)
            n86 = call "replace cursor - plot ref - V2.vi"("Plot ref in"=w125, "new X"=w128, "new  Y"=w129, "cursor index"=4, "cursor action"=cursor_action."write") -> ()  [unwired: 11 in, 4 out]
            n87 = local write "phase0"(w130) -> ()
            n88 = local write "phase"(w130) -> ()
          }
          frame "action: update hist from omega" {
            n89 = call "replace cursor - plot ref - V2.vi"("Plot ref in"=w150, "cursor index"=0, "cursor action"=cursor_action."read") -> ("read X"=w158:dbl, "read Y"=w157:dbl)  [unwired: 13 in, 2 out]
            n90 = Re/Im To Complex(1:w157, 2:w158) -> (0:w159:cdb)
            n91 = local read "factor"() -> (w148:dbl)
            n92 = local read "phase0"() -> (w149:dbl)
            n93 = local read "lorentzian"() -> (w147:T1)
            n94 = local read "omega"() -> (w156:dbl)
            n95 = Add(x=w149, y=0.01) -> (x+y=w146:dbl)
            n96 = Generate User Event(user event=w151, event data cluster="action: update circle" ("event data")) -> ()  [unwired: 2 in, 2 out]
            n97 = call "lorentzian transformations.vi"("factor"=w148, "4 corner circle transformation"=four-corner_circle_transformation."get f0 given f and phi", "lorentzian in"=w147, "phase in (rad)"=w146, "freq in"=w156, "voltage in"=w159) -> ("lorentzian out"=w160:T1)  [unwired: 2 in, 3 out]
            n98 = local write "lorentzian hist"(w160) -> ()
          }
        }
      }
    }
  }
